vi "test.vi"(8 "error in (no error)":errorcluster, 11 "Autofocus in":refnum<class "Autofocus.lvclass">) -> (0 "error out":errorcluster, 3 "Autofocus out":refnum<class "Autofocus.lvclass">)   [LabVIEW 2012, in "Autofocus.lvclass"]
uses:
  Autofocus.lvclass
  Sharpness Measure.ctl
  Autofocus.lvclass/Autofocus.ctl
  <vilib>/Utility/file.llb/Write To Spreadsheet File (DBL).vi
  <vilib>/Utility/file.llb/Write To Spreadsheet File (string).vi
panel:
  in  "Image to select ROI":path
  in  "ROI?":bool
  out "Image Source":T1(plugin-control)
  out "Number of Files found in fodler":i32
  out "Array":dbl[](array[numeric])
  in  "File Path":path
  in  "Sharpness measure":T2
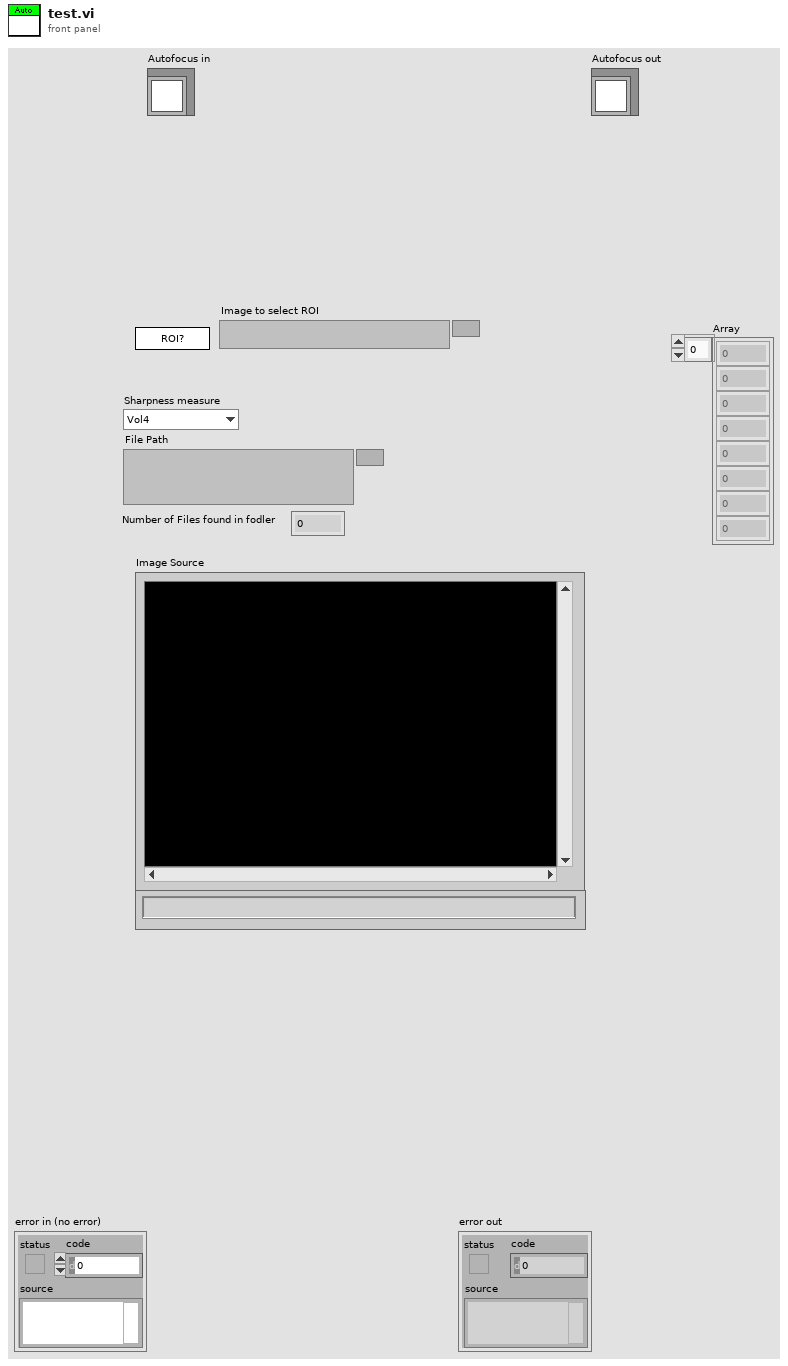
[diagram p1: front panel]
types:
  T1 = typedef "IMAQ Image.ctl" = refnum<image>
  T2 = typedef "Autofocus.lvclass/Sharpness Measure.ctl" = enum16{"Vol4", "Gradient Square"}
  T3 = typedef "Image Type" = u32
  T4 = typedef "ROI Descriptor" = cluster{"Global Rectangle":i32[], "Contours":cluster{"ID":enum32{"External", "Internal"}, "Type":u32, "Coordinates":i32[]}[]}
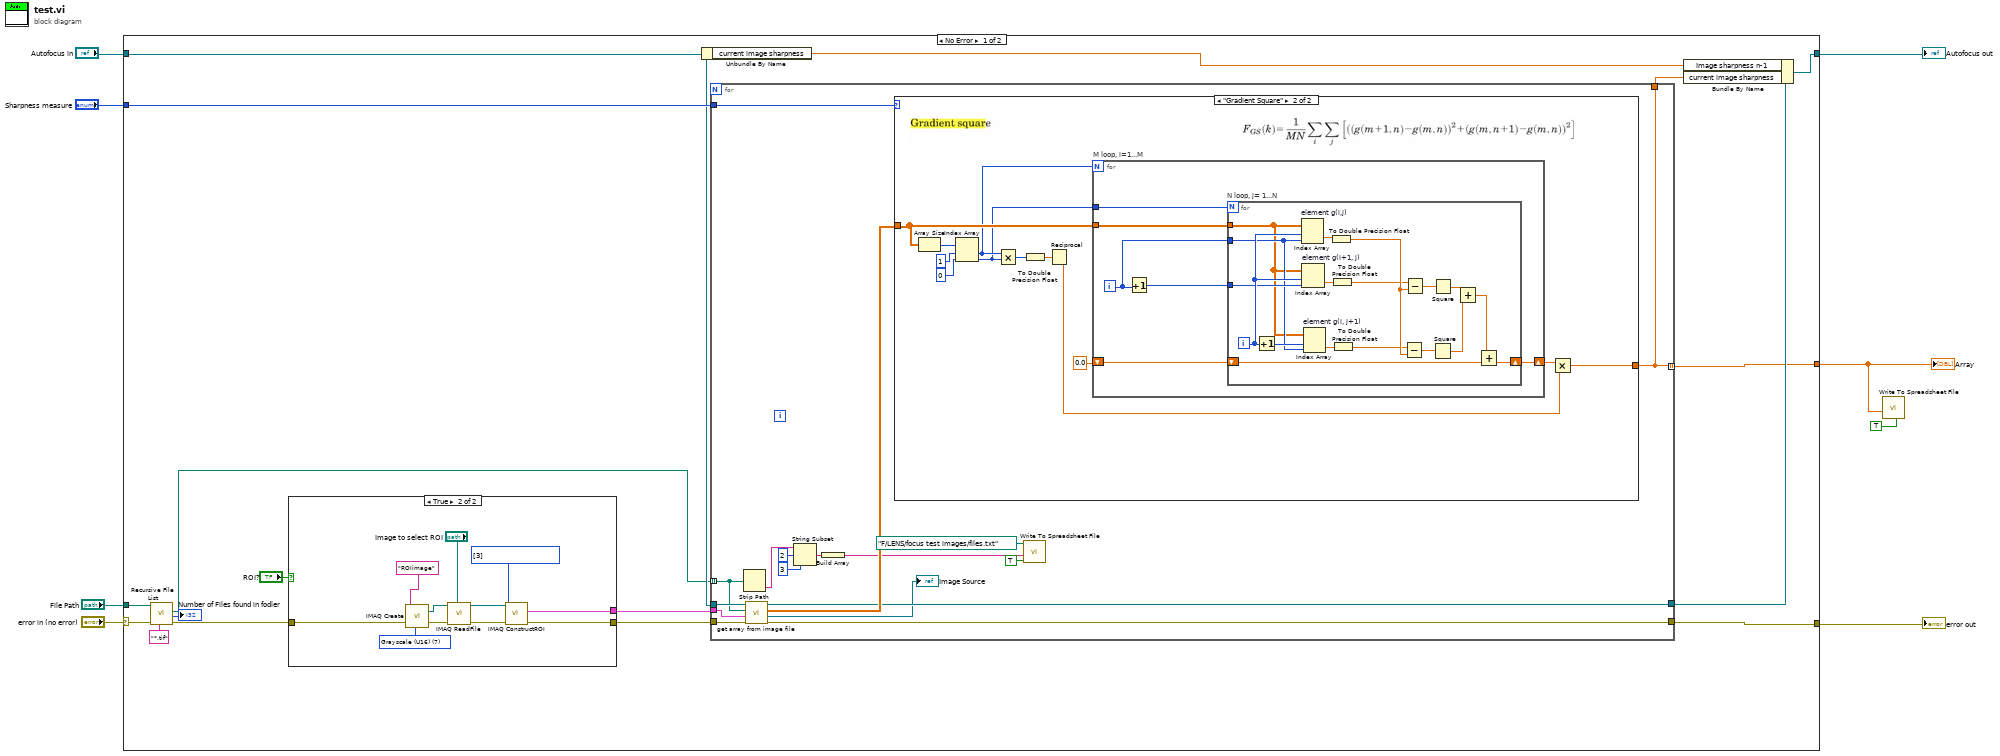
[diagram p0: block diagram]
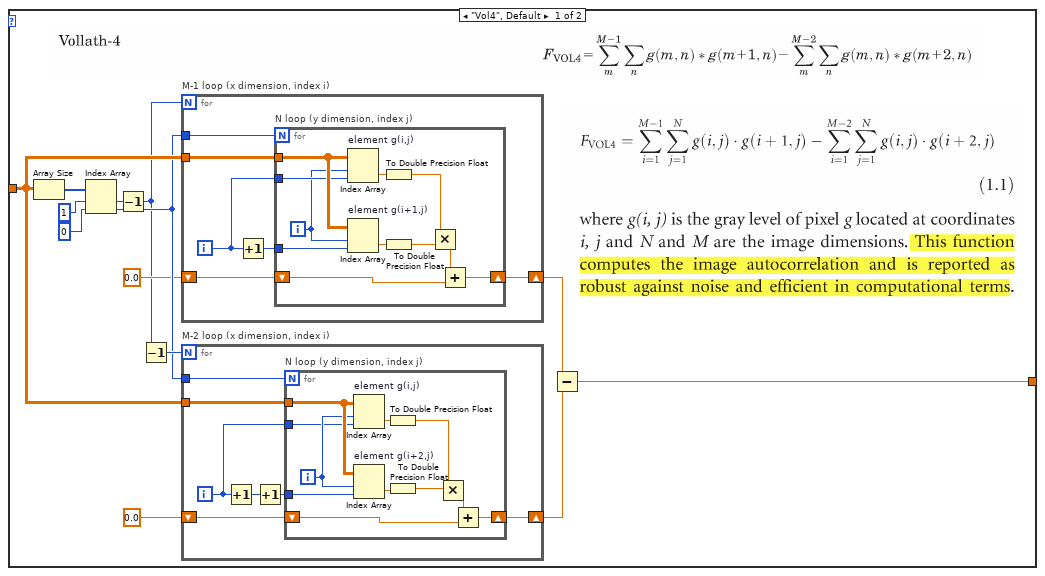
[diagram p3: hidden frame]
diagram:
  n1 = case shown="No Error" "error in (no error)" {
    selector: "error in (no error)" -> [w19 w140]
    tunnel: [w23 w140] -> w7
    tunnel: [w20 w139] -> w5
    tunnel: "Autofocus in" -> [w22 w139]
    tunnel: "Sharpness measure" -> [w24 _]
    tunnel: "File Path" -> [w18 _]
    tunnel: [w15 _] -> w2
    frame No Error {
      n2 = call <vilib>:"Recursive File List.vi"("pattern"="*.tif", "error in (no error)"=w19, "Folder Path"=w18) -> ("error out"=w13:errorcluster, "Number of Files"=→"Number of Files found in fodler":i32, "All Files in Dir"=w10:path[])  [unwired: 4 in, 2 out]
      n3 = case shown="True" "ROI?" {
        tunnel: w13 -> [w26 w37]
        tunnel: [w26 w36] -> w12
        tunnel: [_ w35] -> w11
        frame False {
        }
        frame True {
          w32 = T3 7 items=["Grayscale (U8)", "Grayscale (I16)", "Grayscale (SGL)", "Complex (CSG)", "RGB (U32)", "HSL (U32)", "RGB (U64)", "Grayscale (U16)"] ("Image Type")
          w34 = u32[] [3] items=["No Selection", "Point", "Line", "Rectangle", "Oval", "Polygon", "Freehand Region", "Annulus", "Zoom", "Pan", "Broken Line", "Freehand Line", "Rotated Rectangle"] ("Tools")
          n4 = call "IMAQ Create"("Image Name"="ROIimage", "Image Type"=w32, "error in (no error)"=w37) -> ("New Image"=w33:T1, "error out"=w30:errorcluster)  [unwired: 2 in]
          n5 = call "IMAQ ReadFile"("File Path"="Image to select ROI", "error in (no error)"=w30, "Image"=w33) -> ("error out"=w29:errorcluster, "Image Out"=w28:T1)  [unwired: 4 in, 3 out]
          n6 = call "IMAQ ConstructROI"("error in (no error)"=w29, "Tools"=w34, "Image"=w28) -> ("error out"=w36:errorcluster, "ROI Descriptor Out"=w35:T4)  [unwired: 5 in, 2 out]
        }
      }
      n7 = Unbundle By Name(w22) -> ("current image sharpness"=w25:dbl)
      n8 = for {
        tunnel: [w48] -> w16
        tunnel: w24 -> [w54]
        tunnel: w12 -> [w53]
        tunnel: [w52] -> w23
        tunnel: w22 -> [w50]
        tunnel: [w49] -> w21
        tunnel: w10 -> [w45] mode=indexing
        tunnel: [w48] -> w15 mode=indexing
        tunnel: w11 -> [w38]
        n9 = Strip Path(path=w45) -> (name=w43:string)  [unwired: 1 out]
        n10 = call-dynamic "get array from image file.vi"("error in (no error)"=w53, "ROI Descriptor Out"=w38, "File Path"=w45, "Autofocus in"=w50) -> ("error out"=w52:errorcluster, "Image Source"=→"Image Source":T1, "Array"=w51:dbl[][], "Autofocus out"=w49:refnum<class "Autofocus.lvclass">)  [unwired: 4 in]
        n11 = String Subset(string=w43, offset (0)=2, length (rest)=3 ("length (rest)")) -> (substring=w42:string)
        n12 = Build Array(w42) -> (w44:string[])
        n13 = case shown="\"Gradient Square\"" w54 {
          tunnel: w51 -> [w62 w111]
          tunnel: [w56 w106] -> w48
          frame "Vol4", Default {
            n14 = Array Size(array=w62) -> (size(s)=w67:i32[])
            n15 = Index Array(array=w67, index #1=1 ("index"), index #2=0 ("index")) -> (element #1=w63:i32, element #2=w61:i32)
            n16 = Decrement(x=w63) -> (x-1=w55:i32)
            n17 = Decrement(x=w55) -> (x-1=w64:i32)
            n18 = for "M-1 loop (x dimension, index i)" {
              N: w55 -> [_]
              tunnel: w62 -> [w91]
              tunnel: w61 -> [w90]
              shift-right: [w87] -> w60
              shift-left: 0.0 -> [w86]
              i -> [w89]
              n19 = Increment(x=w89) -> (x+1=w88:i32)
              n20 = for "N loop (y dimension, index j)" {
                N: w90 -> [_]
                tunnel: w91 -> [w101]
                shift-right: [w94] -> w87
                shift-left: w86 -> [w102]
                tunnel: w89 -> [w99]
                tunnel: w88 -> [w97]
                i -> [w98]
                n21 = Index Array "element g(i,j)"(array=w101, index (row)=w98, index (col)=w99) -> (element=w96:dbl)
                n22 = Index Array "element g(i+1,j)"(array=w101, index (row)=w98, index (col)=w97) -> (element=w95:dbl)
                n23 = To Double Precision Float(number=w96) -> (double precision float=w92:dbl)
                n24 = To Double Precision Float(number=w95) -> (double precision float=w93:dbl)
                n25 = Multiply(x=w92, y=w93) -> (x*y=w100:dbl)
                n26 = Add(x=w100, y=w102) -> (x+y=w94:dbl)
              }
            }
            n27 = for "M-2 loop (x dimension, index i)" {
              N: w64 -> [_]
              tunnel: w62 -> [w73]
              tunnel: w61 -> [w74]
              shift-right: [w69] -> w59
              shift-left: 0.0 -> [w68]
              i -> [w72]
              n28 = Increment(x=w72) -> (x+1=w71:i32)
              n29 = Increment(x=w71) -> (x+1=w70:i32)
              n30 = for "N loop (y dimension, index j)" {
                N: w74 -> [_]
                tunnel: w73 -> [w82]
                tunnel: w72 -> [w80]
                tunnel: w70 -> [w79]
                shift-right: [w78] -> w69
                shift-left: w68 -> [w77]
                i -> [w81]
                n31 = Index Array "element g(i,j)"(array=w82, index (row)=w81, index (col)=w80) -> (element=w84:dbl)
                n32 = Index Array "element g(i+2,j)"(array=w82, index (row)=w81, index (col)=w79) -> (element=w85:dbl)
                n33 = To Double Precision Float(number=w84) -> (double precision float=w75:dbl)
                n34 = To Double Precision Float(number=w85) -> (double precision float=w76:dbl)
                n35 = Multiply(x=w75, y=w76) -> (x*y=w83:dbl)
                n36 = Add(x=w83, y=w77) -> (x+y=w78:dbl)
              }
            }
            n37 = Subtract(x=w60, y=w59) -> (x-y=w56:dbl)
          }
          frame "Gradient Square" {
            n38 = Array Size(array=w111) -> (size(s)=w114:i32[])
            n39 = Index Array(array=w114, index #1=1 ("index"), index #2=0 ("index")) -> (element #1=w104:i32, element #2=w103:i32)
            n40 = Multiply(x=w104, y=w103) -> (x*y=w110:i32)
            n41 = To Double Precision Float(number=w110) -> (double precision float=w109:dbl)
            n42 = Reciprocal(x=w109) -> (1/x=w105:dbl)
            n43 = for "M loop, i=1...M" {
              N: w104 -> [_]
              tunnel: w111 -> [w120]
              tunnel: w103 -> [w119]
              shift-right: [w116] -> w107
              shift-left: 0.0 -> [w115]
              i -> [w118]
              n44 = Increment(x=w118) -> (x+1=w117:i32)
              n45 = for "N loop, j= 1...N" {
                N: w119 -> [_]
                tunnel: w120 -> [w134]
                tunnel: w118 -> [w135]
                tunnel: w117 -> [w137]
                shift-right: [w124] -> w116
                shift-left: w115 -> [w126]
                i -> [w138]
                n46 = Increment(x=w138) -> (x+1=w136:i32)
                n47 = Index Array "element g(i,j)"(array=w134, index (row)=w138, index (col)=w135) -> (element=w129:dbl)
                n48 = Index Array "element g(i+1, j)"(array=w134, index (row)=w138, index (col)=w137) -> (element=w133:dbl)
                n49 = Index Array "element g(i, j+1)"(array=w134, index (row)=w136, index (col)=w135) -> (element=w130:dbl)
                n50 = To Double Precision Float(number=w129) -> (double precision float=w123:dbl)
                n51 = To Double Precision Float(number=w133) -> (double precision float=w122:dbl)
                n52 = To Double Precision Float(number=w130) -> (double precision float=w121:dbl)
                n53 = Subtract(x=w121, y=w123) -> (x-y=w131:dbl)
                n54 = Subtract(x=w122, y=w123) -> (x-y=w132:dbl)
                n55 = Square(x=w131) -> (x^2=w127:dbl)
                n56 = Square(x=w132) -> (x^2=w128:dbl)
                n57 = Add(x=w128, y=w127) -> (x+y=w125:dbl)
                n58 = Add(x=w125, y=w126) -> (x+y=w124:dbl)
              }
            }
            n59 = Multiply(x=w107, y=w105) -> (x*y=w106:dbl)
          }
        }
        n60 = call-poly <vilib>:"Write To Spreadsheet File.vi"("append to file? (new file:F)"=TRUE, "1D data"=w44, "file path (dialog if empty)"=path "F:/LENS/focus test images/files.txt") -> ()  [unwired: 5 in, 1 out]
      }
      n61 = Bundle By Name(cluster=w21, "Image sharpness n-1"=w25, "current image sharpness"=w16) -> (w20:refnum<class "Autofocus.lvclass">)
    }
    frame Error {
    }
  }
  "error out" <- w7
  "Autofocus out" <- w5
  "Array" <- w2
  n62 = call-poly <vilib>:"Write To Spreadsheet File.vi"("transpose? (no:F)"=TRUE, "1D data"=w2) -> ()  [unwired: 6 in, 1 out]
